vi "Generate Neopixel RT DVR.vi"(8 "Error In":errorcluster, 11 "Display In":refnum<class "Neopixel - Host.lvclass">) -> (0 "Error Out":errorcluster, 3 "Display Out":refnum<class "Neopixel - Host.lvclass">)   [LabVIEW 2021, in "Neopixel - Host.lvclass"]
uses:
  Neopixel - Host.lvclass
  Controls/Data.ctl
  Public/Controls/FPGA Reference.ctl
  Public/Controls/RGB Gains.ctl
  Neopixel - Host.lvclass/Neopixel - Host.ctl
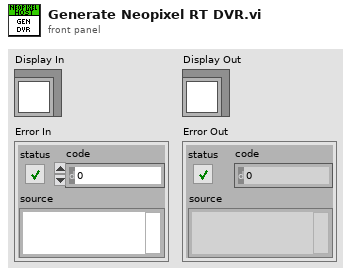
[diagram p1: front panel]
types:
  T1 = typedef "Neopixel - Host.lvclass/Data.ctl" = cluster{"FPGA VI Reference":T2, "RGB Gains":T3}
  T2 = typedef "Neopixel - Host.lvclass/FPGA Reference.ctl" = refnum<k20>
  T3 = typedef "Neopixel - Host.lvclass/RGB Gains.ctl" = cluster{"Red":sgl, "Green":sgl, "Blue":sgl}
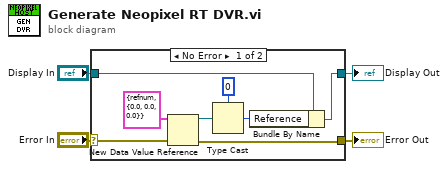
[diagram p0: block diagram]
diagram:
  n1 = case shown="No Error" "Error In" {
    selector: "Error In" -> [w11 w14]
    tunnel: "Display In" -> [w8 w13]
    tunnel: [w5 w14] -> w2
    tunnel: [w6 w13] -> w1
    frame No Error {
      n2 = New Data Value Reference(data value=T1 {"FPGA VI Reference"=refnum, "RGB Gains"={"Red"=0.0, "Green"=0.0, "Blue"=0.0}} ("Data"), error in=w11) -> (data value reference=w9:refnum<data-value>, error out=w5:errorcluster)
      n3 = Type Cast(type=u64 0, x=w9) -> (*(type *) &x=w7:u64)
      n4 = Bundle By Name(cluster=w8, "Reference"=w7) -> (w6:refnum<class "Neopixel - Host.lvclass">)
    }
    frame Error {
    }
  }
  "Display Out" <- w1
  "Error Out" <- w2
